vi "QR Reader.vi"(8 "error in (no error)":errorcluster, 11 "Image Filepath":path) -> (0 "error out":errorcluster)   [LabVIEW 2014]
uses:
  <vilib>/Platform/browser.llb/Open URL in Default Browser (string).vi
panel:
  in  "Launch Browser (F)":bool
  in  "Draw Green Square (F)":bool
  out "Barcode Data":string
  out "Image Display":T1(plugin-control)
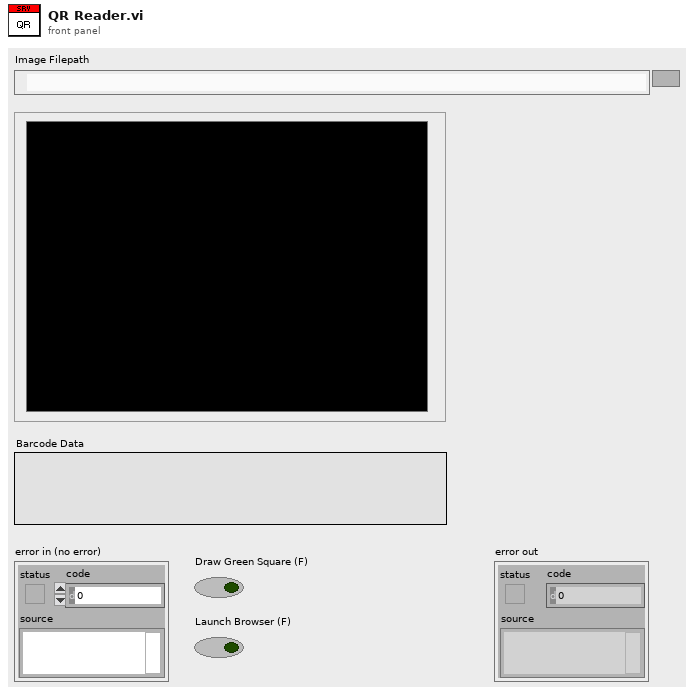
[diagram p1: front panel]
types:
  T1 = typedef "IMAQ Image.ctl" = refnum<image>
  T2 = typedef "QR Code Report.ctl" = cluster{"Found?":bool, "Data":string, "Bounding Box":cluster{"x":sgl, "y":sgl}[], "Errors Corrected":u32, "Dimensions (Rows/Cols)":u32, "Version":u32, "QR Model":T3, "Stream Mode":T4, "Barcode Polarity":T5, "Mirrored?":bool, "Append Stream Position":u32, "Size of Append Stream":u32, "First EAN-128 ID":i32, "First Alternate Language ID":i32, "Append Stream ID":u32, "Minimum Edge Strength":u32, "Demodulation Mode":T6, "Cell Sample Size":T7, "Cell Filter Mode":T8}
  T3 = typedef "QR Code Model Type.ctl" = i32
  T4 = typedef "QR Code Stream Mode Type.ctl" = i32
  T5 = typedef "Data Matrix Polarity.ctl" = i32
  T6 = typedef "Demodulation Mode.ctl" = i32
  T7 = typedef "Cell Sample Size.ctl" = i32
  T8 = typedef "Cell Filter Mode.ctl" = i32
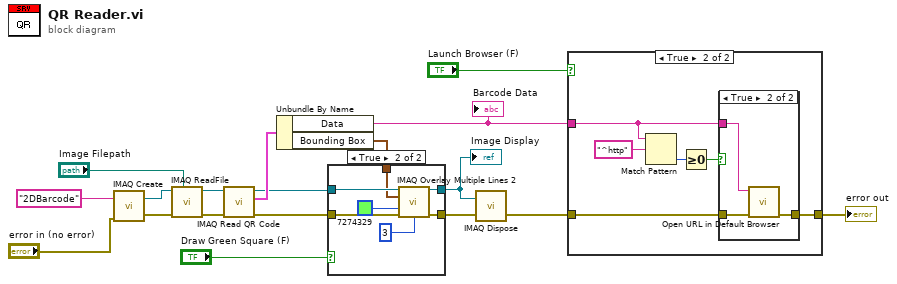
[diagram p0: block diagram]
diagram:
  n1 = call "IMAQ Create"("Image Name"="2DBarcode", "error in (no error)"="error in (no error)") -> ("New Image"=w18:T1, "error out"=w17:errorcluster)  [unwired: 3 in]
  n2 = call "IMAQ ReadFile"("File Path"="Image Filepath", "error in (no error)"=w17, "Image"=w18) -> ("error out"=w13:errorcluster, "Image Out"=w14:T1)  [unwired: 4 in, 3 out]
  n3 = call "IMAQ Read QR Code"("error in (no error)"=w13, "Image"=w14) -> ("error out"=w9:errorcluster, "QR Code Report"=w15:T2, "Image (duplicate)"=w12:T1)  [unwired: 6 in, 1 out]
  n4 = Unbundle By Name(w15) -> ("Data"=w6:string, "Bounding Box"=w11:cluster{"x":sgl, "y":sgl}[])
  "Barcode Data" <- w6
  n5 = case shown="True" "Draw Green Square (F)" {
    tunnel: w12 -> [w19 w27]
    tunnel: w11 -> [_ w26]
    tunnel: [w20 w24] -> w10
    tunnel: w9 -> [w20 w23]
    tunnel: [w19 w21] -> w8
    frame False {
    }
    frame True {
      n6 = call "IMAQ Overlay Multiple Lines 2"("Image"=w27, "Line End Points"=w26, "Color"=u32 7274329, "error in (no error)"=w23, "Width"=u32 3) -> ("Image Out"=w21:T1, "error out"=w24:errorcluster)  [unwired: 9 in]
    }
  }
  "Image Display" <- w8
  n7 = call "IMAQ Dispose"("Image"=w8, "error in (no error)"=w10) -> ("error out"=w7:errorcluster)  [unwired: 4 in]
  n8 = case shown="True" "Launch Browser (F)" {
    tunnel: w7 -> [w28 w34]
    tunnel: w6 -> [_ w31]
    tunnel: [w28 w33] -> w3
    frame False {
    }
    frame True {
      n9 = Match Pattern(string=w31, regular expression="^http") -> (offset past match=w30:i32)  [unwired: 1 in, 3 out]
      n10 = Greater Or Equal To 0?(x=w30) -> (x >= 0?=w29:bool)
      n11 = case shown="True" w29 {
        tunnel: w34 -> [w35 w38]
        tunnel: w31 -> [_ w37]
        tunnel: [w35 w36] -> w33
        frame False {
        }
        frame True {
          n12 = call-poly <vilib>:"Open URL in Default Browser.vi"("error in (no error)"=w38, "URL"=w37) -> ("error out"=w36:errorcluster)  [unwired: 4 in, 1 out]
        }
      }
    }
  }
  "error out" <- w3
